vi "string_cut.vi"(8 "error in (no error)":errorcluster caption="에러 입력(에러 없음)", 10 "종료문자":string="?", 11 "수신문자열":string) -> (0 "error out":errorcluster caption="에러 출력", 2 "나머지문자열":string, 3 "완성문자열":string)   [LabVIEW 2014]
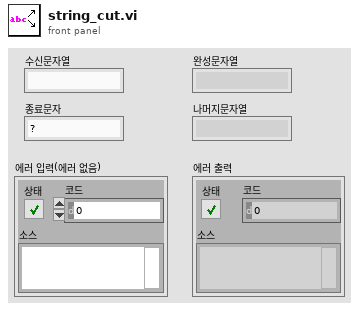
[diagram p1: front panel]
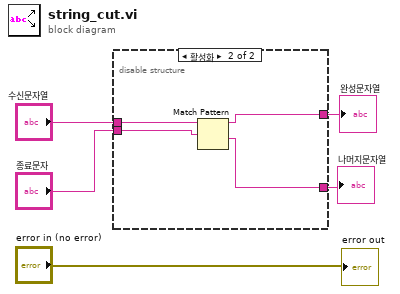
[diagram p0: block diagram]
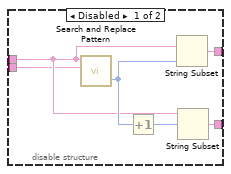
[diagram p2: hidden frame]
diagram:
  n1 = disable-structure shown="활성화" {
    disable-tunnel: [w11 w12] -> w5
    disable-tunnel: [w10 w13] -> w4
    disable-tunnel: "수신문자열" -> [w7 w15]
    disable-tunnel: "종료문자" -> [w6 w14]
    frame Disabled {
      n2 = call <vilib>:"Search and Replace Pattern.vi"("string"=w7, "regular expression (\"\")"=w6) -> ("offset past match"=w9:i32)  [unwired: 3 in, 1 out]
      n3 = Increment(x=w9) -> (x+1=w8:i32)
      n4 = String Subset(string=w7, length (rest)=w9) -> (substring=w11:string)  [unwired: 1 in]
      n5 = String Subset(string=w7, offset (0)=w8) -> (substring=w10:string)  [unwired: 1 in]
    }
    frame Enabled {
      n6 = Match Pattern(string=w15, regular expression=w14) -> (before substring=w12:string, after substring=w13:string)  [unwired: 1 in, 2 out]
    }
  }
  "완성문자열" <- w5
  "나머지문자열" <- w4
  "error out" <- "error in (no error)"
